vi "TimeoutParse_SubVI.vi"(8 "error in (no error)":errorcluster) -> (0 "error out":errorcluster, 3 "Connected?":bool)   [LabVIEW 2017]
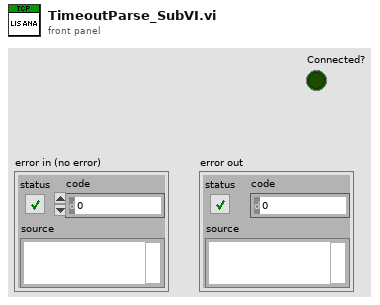
[diagram p1: front panel]
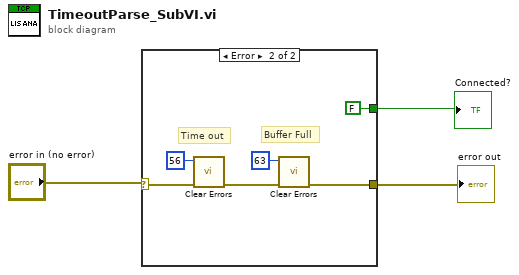
[diagram p0: block diagram]
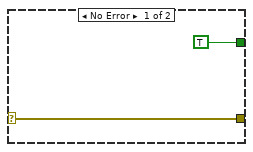
[diagram p2: hidden frame]
diagram:
  n1 = case shown="Error" "error in (no error)" {
    selector: "error in (no error)" -> [w5 w10]
    tunnel: [w5 w7] -> w3
    tunnel: [TRUE ("Connected") FALSE ("Connected")] -> w1
    frame No Error {
    }
    frame Error {
      # "Buffer Full"
      # "Time out"
      n2 = call <vilib>:"Clear Errors.vi"("error in (no error)"=w10, "specific error code to clear (0: all)"=56) -> ("error out"=w8:errorcluster)  [unwired: 4 in, 1 out]
      n3 = call <vilib>:"Clear Errors.vi"("error in (no error)"=w8, "specific error code to clear (0: all)"=63) -> ("error out"=w7:errorcluster)  [unwired: 4 in, 1 out]
    }
  }
  "error out" <- w3
  "Connected?" <- w1
